vi "RadToDeg.vi"(1 "rad":dbl) -> (0 "deg":dbl)   [LabVIEW 2018]
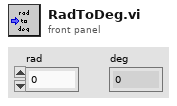
[diagram p1: front panel]
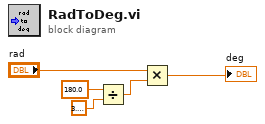
[diagram p0: block diagram]
diagram:
  n1 = Divide(x=180.0, y=3.141592653589793) -> (x/y=w3:dbl)
  n2 = Multiply(x="rad", y=w3) -> (x*y=→"deg":dbl)
